vi "AnyBuilderBuild.vi"(8 "error in (no error)":errorcluster, 10 "Message Type":string, 11 "Builder Ref":T2) -> (0 "error out":errorcluster, 3 "Any":T1)   [LabVIEW 2019, in "gprc-lvsupport.lvlib"]
uses:
  gprc-lvsupport.lvlib
  typeDefs/Any.ctl
  typeDefs/grpcId.ctl
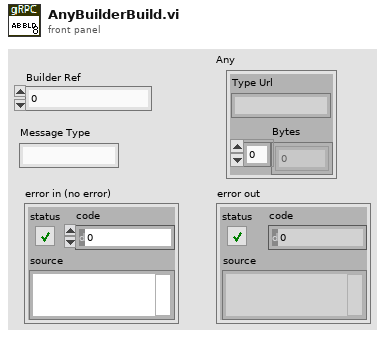
[diagram p1: front panel]
types:
  T1 = typedef "gprc-lvsupport.lvlib/Any.ctl" = cluster{"Type Url":string, "Bytes":u8[]}
  T2 = typedef "gprc-lvsupport.lvlib/grpcId.ctl" = u64
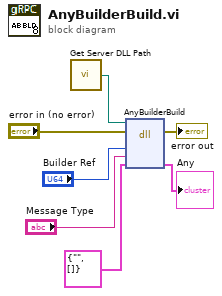
[diagram p0: block diagram]
diagram:
  n1 = call "Get Server DLL Path.vi"() -> ("Server dll path"=w6:path)
  n2 = dll-call lib="?" fn="AnyBuilderBuild"(path in=w6, error in="error in (no error)", "builderId"="Builder Ref", "messageType"="Message Type", "any"=T1 {"Type Url"="", "Bytes"=[]} ("Any")) -> (error out=→"error out":errorcluster, "any"=→"Any":T1)  [unwired: 4 in, 1 out]
